vi "TETRIX WatchDog_HT_myRIO.vi"(3 "error in (no error)":errorcluster) -> (1 "error out":errorcluster)   [LabVIEW 2013]
uses:
  <vilib>/Platform/TimedLoop/XDataNode/timing_clust.ctl
  <vilib>/Platform/TimedLoop/XDataNode/nitl_modes.ctl
  <vilib>/Platform/TimedLoop/XDataNode/wakeup.ctl
  <vilib>/myRIO/Instrument Drivers/Onboard IO/I2C/vis/Smart Open.vi
  <vilib>/myRIO/Instrument Drivers/Onboard IO/I2C/vis/Configure.vi
  <vilib>/myRIO/Instrument Drivers/Onboard IO/I2C/vis/Write.vi
  <vilib>/myRIO/Instrument Drivers/Onboard IO/I2C/vis/Open.vi
  <vilib>/myRIO/Common/Instrument Driver Framework/myRIO v1.0/I2C/vis/myRIO v1.1 Open I2C.vi
  <vilib>/myRIO/Common/Instrument Driver Framework/Utilities/vis/Validate Channels.vi
  <vilib>/myRIO/Common/Instrument Driver Framework/myRIO v1.0/I2C/vis/myRIO v1.0 Reserve I2C.vi
  <vilib>/myRIO/Common/Instrument Driver Framework/myRIO v1.0/I2C/vis/myRIO v1.0 Build MUX Configuration I2C.vi
  <vilib>/myRIO/Common/Instrument Driver Framework/myRIO v1.0/Resource Manager/vis/myRIO v1.0 Reserve Channel List.vi
  <vilib>/myRIO/Common/Instrument Driver Framework/myRIO v1.0/Resource Manager/vis/myRIO v1.0 Create Configuration List.vi
  <vilib>/myRIO/Common/Instrument Driver Framework/myRIO v1.0/Resource Manager/vis/myRIO v1.0 Reserve Channel.vi
  <vilib>/myRIO/Common/Instrument Driver Framework/myRIO v1.0/Resource Manager/vis/myRIO v1.0 Unreserve Channel.vi
  <vilib>/myRIO/Common/Instrument Driver Framework/myRIO v1.0/Resource Manager/vis/myRIO v1.0 Build Mutex Name.vi
  <vilib>/myRIO/Common/Instrument Driver Framework/myRIO v1.0/myRIO v1.1 Open.vi
  <vilib>/Utility/VariantDataType/GetNumericInfo.vi
  <vilib>/Utility/error.llb/Error Cluster From Error Code.vi
  <vilib>/myRIO/Common/Instrument Driver Framework/Utilities/vis/IO Manager.vi
  <vilib>/myRIO/Common/Instrument Driver Framework/Utilities/vis/Configuration Manager.vi
  <vilib>/myRIO/Common/Instrument Driver Framework/myRIO v1.0/Resource Manager/vis/myRIO v1.0 Configure IO.vi
  <vilib>/myRIO/Common/Instrument Driver Framework/myRIO v1.0/myRIO v1.0 Close.vi
  <vilib>/myRIO/Common/Instrument Driver Framework/myRIO v1.0/I2C/vis/myRIO v1.0 Configure I2C.vi
  <vilib>/myRIO/Common/Instrument Driver Framework/myRIO v1.0/I2C/vis/myRIO v1.0 Write I2C.vi
  <vilib>/platform/TimedLoop/XDataNode/XDataNode.xnode
  <vilib>/Platform/TimedLoop/XDataNode/XDNodeRunTimeDep.lvlib
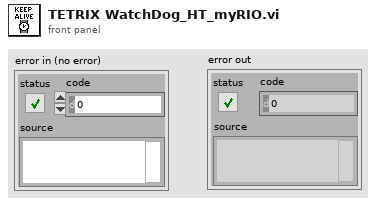
[diagram p1: front panel]
types:
  T1 = typedef "XDNodeRunTimeDep.lvlib/timing_clust.ctl" = cluster{"Expected End [f-1]":u64, "Actual End [f-1]":u64, "Finished Late? [f-1]":bool, "Expected End [i-1]":u64, "Actual End [i-1]":u64, "Finished Late? [i-1]":bool, "Expected Start [i]":u64, "Actual Start [i]":u64, "Expected Start [f]":u64, "Actual Start [f]":u64, "Source Name":string, "Structure Name":string, "Period":i64, "Deadline":i64, "Offset":i64, "Start":i64, "Priority":i32, "Timeout":i32, "Mode":T2, "Wakeup Reason":T3, "Error":errorcluster, "Source Type":string, "Secondary Source Type":string, "Global End Time":u64, "Global Start Time":u64, "Frame Duration":u64, "Iteration Duration":u64, "Assigned CPU":i32, "I/O Scan Engine Mode":u32}
  T2 = typedef "XDNodeRunTimeDep.lvlib/nitl_modes.ctl" = enum32{"No Change", "Process missed periods, maintain original phase", "Discard missed periods, maintain original phase", "Process missed periods, ignore original phase", "Discard missed periods, ignore original phase"}
  T3 = typedef "XDNodeRunTimeDep.lvlib/wakeup.ctl" = enum32{"Normal", "Aborted", "Asynchronous wakeup", "Timing source error", "Timed loop error", "Timeout"}
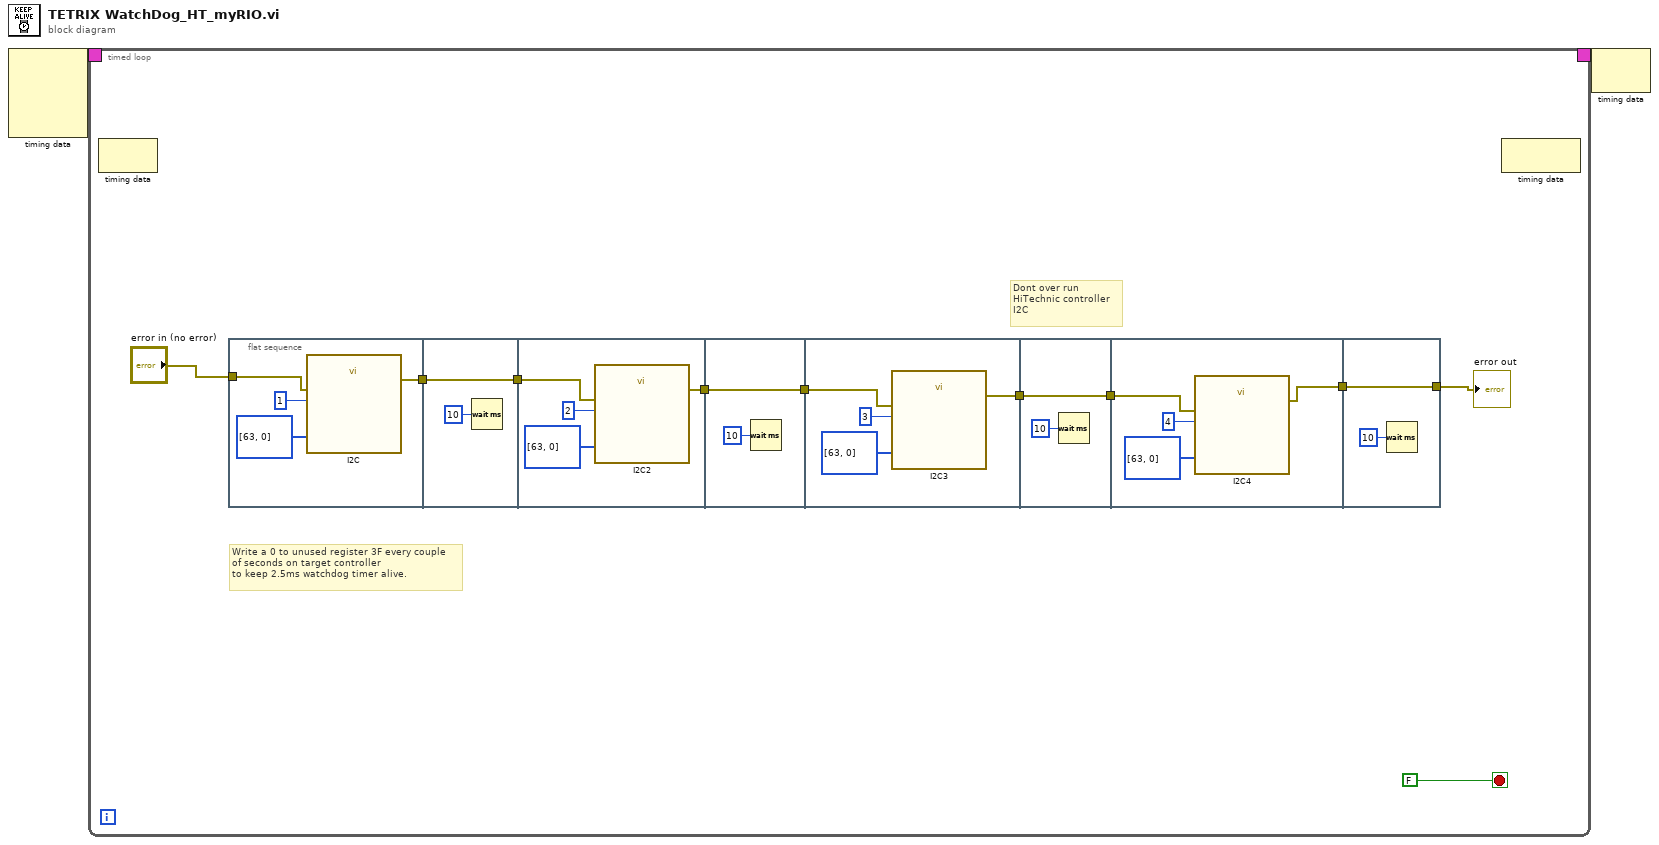
[diagram p0: block diagram]
diagram:
  n1 = node-c288() -> (w2:T1)  [unwired: 4 in]
  n2 = timed-loop {
    timing: w2 -> [_]
    timing-out: [_] -> w1
    stop <- FALSE stop-if-true
    # "Dont over run\nHiTechnic controller\nI2C"
    # "Write a 0 to unused register 3F every couple\nof seconds on target controller\nto keep 2.5ms watchdog timer alive."
    n3 = node-c288() -> ()  [unwired: 1 in, 1 out]
    n4 = flat-sequence {
      tunnel: "error in (no error)" -> [w14]
      tunnel: [w13] -> w11
      tunnel: [w17] -> w10
      tunnel: w11 -> [w17]
      tunnel: w10 -> [w20]
      tunnel: [w19] -> w9
      tunnel: [w23] -> w8
      tunnel: w9 -> [w23]
      tunnel: w8 -> [w26]
      tunnel: [w25] -> w7
      tunnel: [w29] -> w6
      tunnel: w7 -> [w29]
      tunnel: w6 -> [w32]
      tunnel: [w31] -> w5
      tunnel: [w36] -> w3
      tunnel: w5 -> [w36]
      frame #0 {
        n5 = call "I2C"("Slave Address (7-bit)"=u8 1, "Bytes to Write"=u8[] [63, 0], "error in (no error)"=w14) -> ("error out"=w13:errorcluster)  [unwired: 24 in]
      }
      frame #1 {
        n6 = Wait (ms)(milliseconds to wait=u32 10) -> ()  [unwired: 1 out]
      }
      frame #2 {
        n7 = call "I2C2"("Slave Address (7-bit)"=u8 2, "Bytes to Write"=u8[] [63, 0], "error in (no error)"=w20) -> ("error out"=w19:errorcluster)  [unwired: 24 in]
      }
      frame #3 {
        n8 = Wait (ms)(milliseconds to wait=u32 10) -> ()  [unwired: 1 out]
      }
      frame #4 {
        n9 = call "I2C3"("Slave Address (7-bit)"=u8 3, "Bytes to Write"=u8[] [63, 0], "error in (no error)"=w26) -> ("error out"=w25:errorcluster)  [unwired: 24 in]
      }
      frame #5 {
        n10 = Wait (ms)(milliseconds to wait=u32 10) -> ()  [unwired: 1 out]
      }
      frame #6 {
        n11 = call "I2C4"("Slave Address (7-bit)"=u8 4, "Bytes to Write"=u8[] [63, 0], "error in (no error)"=w32) -> ("error out"=w31:errorcluster)  [unwired: 24 in]
      }
      frame #7 {
        n12 = Wait (ms)(milliseconds to wait=u32 10) -> ()  [unwired: 1 out]
      }
    }
    n13 = node-c288() -> ()  [unwired: 1 in, 1 out]
    "error out" <- w3
  }
  n14 = node-c288(w1) -> ()  [unwired: 1 out]
